vi "Configure Setpoint 2.vi"(5 "Retry Attempts (0)":i32 min=0, 7 "Unit Address (-1)":i32=-1, 8 "error in (no error)":errorcluster, 9 "Setpoint Type (deviation)":T1=enum."Deviation", 10 "Setpoint value":dbl format="%#_13g", 11 "VISA resource name (in)":refnum<visa-resource-name>) -> (0 "error out":errorcluster, 2 "Response Cluster":T2 {"Command ID" format="%x"}, 3 "VISA resource name (out)":refnum<visa-resource-name>)   [LabVIEW 2020, in "Omega Platinum Series.lvlib"]
doc: "Configures setpoint 2. This can either be given as a second setpoint, or as a deviation (+/-) of setpoint 1."
uses:
  Omega Platinum Series.lvlib
  Type Defs/Response.ctl
  Type Defs/Setpoint Type.ctl
panel:
  out "Command":string
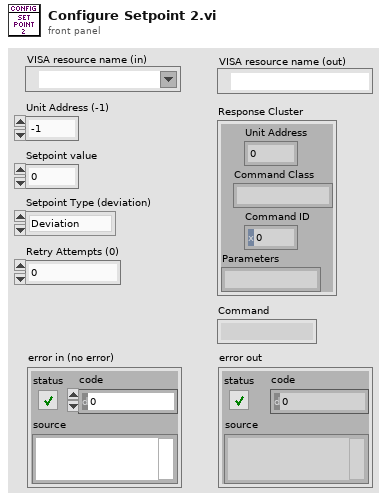
[diagram p1: front panel]
types:
  T1 = typedef "Omega Platinum Series.lvlib/Setpoint Type.ctl" = enum16{"Fixed Constant", "Deviation"}
  T2 = typedef "Omega Platinum Series.lvlib/Response.ctl" = cluster{"Unit Address":i32, "Command Class":string, "Command ID":u32, "Parameters":string}
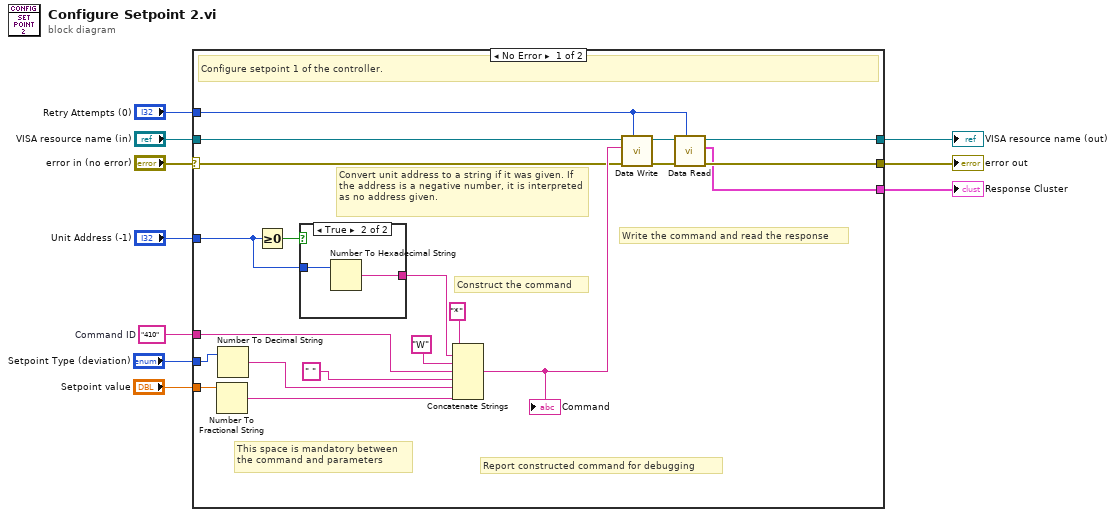
[diagram p0: block diagram]
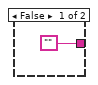
[diagram p2: hidden frame]
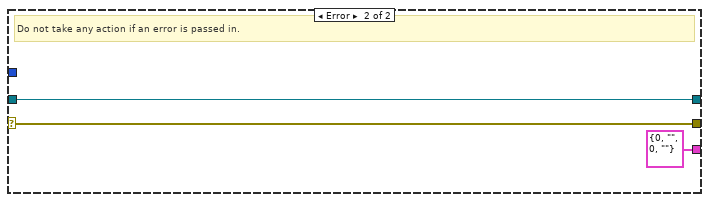
[diagram p3: hidden frame]
diagram:
  w10 = "410"  # Command ID
  n1 = case shown="No Error" "error in (no error)" {
    selector: "error in (no error)" -> [w24 w36]
    tunnel: w10 -> [w14 _]
    tunnel: "Unit Address (-1)" -> [w28 _]
    tunnel: [w20 w36] -> w7
    tunnel: "VISA resource name (in)" -> [w26 w35]
    tunnel: [w21 w35] -> w5
    tunnel: [w19 T2 {"Unit Address"=0, "Command Class"="", "Command ID"=0, "Parameters"=""} ("Response Cluster")] -> w4
    tunnel: "Setpoint value" -> [w16 _]
    tunnel: "Setpoint Type (deviation)" -> [w13 _]
    tunnel: "Retry Attempts (0)" -> [w11 _]
    frame No Error {
      # "Report constructed command for debugging"
      # "Write the command and read the response"
      # "This space is mandatory between\nthe command and parameters"
      # "Convert unit address to a string if it was given. If the address is a negative number, it is interpreted as no address given."
      # "Construct the command"
      # "Configure setpoint 1 of the controller."
      n2 = Number To Fractional String(number=w16) -> (F-format string=w15:string)  [unwired: 3 in]
      n3 = Number To Decimal String(number=w13) -> (decimal integer string=w12:string)  [unwired: 1 in]
      n4 = Greater Or Equal To 0?(x=w28) -> (x >= 0?=w30:bool)
      n5 = case shown="True" w30 {
        tunnel: w28 -> [_ w33]
        tunnel: ["" w32] -> w27
        frame False {
        }
        frame True {
          n6 = Number To Hexadecimal String(2:w33) -> (0:w32:string)  [unwired: 1 in]
        }
      }
      n7 = Concatenate Strings("*" ("string"), w27, "W" ("string"), w14, " " ("string"), w12, w15) -> (w25:string)
      "Command" <- w25
      n8 = call "Data Write.vi"("Retry Attempts (0)"=w11, "error in (no error)"=w24, "Command"=w25, "VISA Refnum in"=w26) -> ("error out"=w23:errorcluster, "VISA Refnum out"=w22:refnum<visa-resource-name>)  [unwired: 6 in]
      n9 = call "Data Read.vi"("Retry Attempts (0)"=w11, "error in (no error)"=w23, "VISA Refnum in"=w22) -> ("error out"=w20:errorcluster, "Response Cluster"=w19:T2, "VISA Refnum out"=w21:refnum<visa-resource-name>)  [unwired: 5 in, 1 out]
    }
    frame Error {
      # "Do not take any action if an error is passed in."
    }
  }
  "error out" <- w7
  "VISA resource name (out)" <- w5
  "Response Cluster" <- w4
